vi "hola mundo.vi"() -> ()   [LabVIEW 2020]
panel:
  in  "String 3":string
  out "String 2":string
  in  "String":string
  out "Boolean 4":bool
  in  "Boolean 3":bool
  in  "Cancel Button":bool
  out "Boolean 2":bool
  in  "Boolean":bool
  out "Indicador D 3":dbl
  in  "Control C 4":dbl
  out "Indicador D 2":dbl
  in  "Control C 3":dbl
  in  "Control C 2":dbl
  out "Indicador D":dbl
  in  "Control C":dbl
  out "Indicador B":i32
  in  "Control A":i32
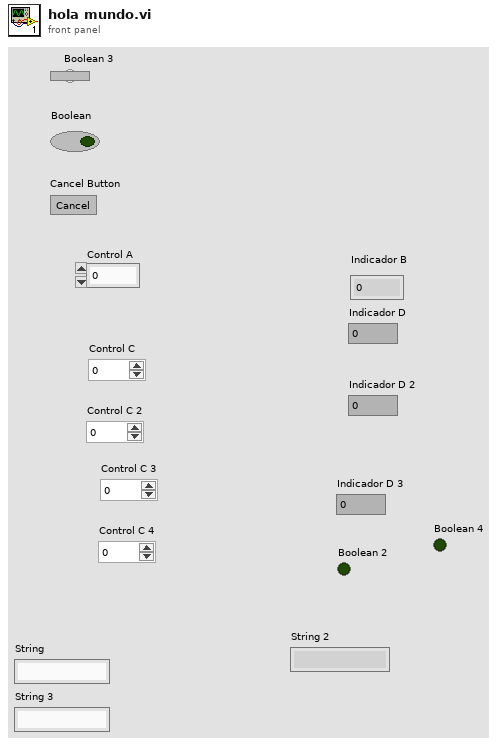
[diagram p1: front panel]
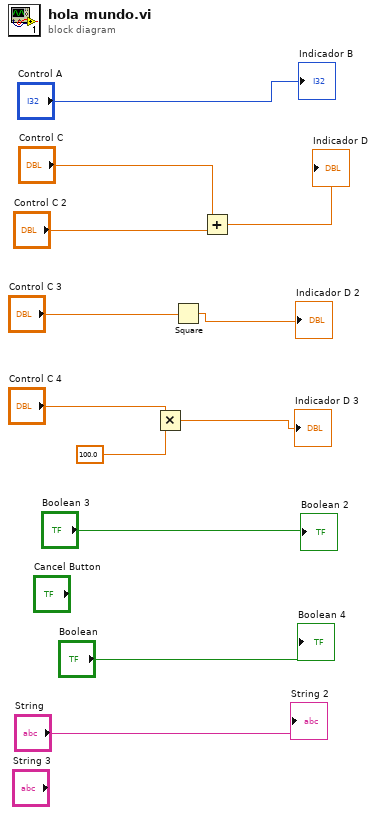
[diagram p0: block diagram]
diagram:
  n1 = Multiply(x="Control C 4", y=100.0) -> (x*y=→"Indicador D 3":dbl)
  n2 = Square(x="Control C 3") -> (x^2=→"Indicador D 2":dbl)
  n3 = Add(x="Control C", y="Control C 2") -> (x+y=→"Indicador D":dbl)
  "Indicador B" <- "Control A"
  "Boolean 2" <- "Boolean 3"
  "Boolean 4" <- "Boolean"
  "String 2" <- "String"
